vi "Global wiggle variables.vi"() -> ()   [LabVIEW 2017]
panel:
  in  "Z frequency":dbl
  in  "Z amplitude":dbl
  in  "Y frequency":dbl
  in  "Y amplitude":dbl
  out "Wiggle stop":bool
  in  "X frequency":dbl
  in  "X amplitude":dbl
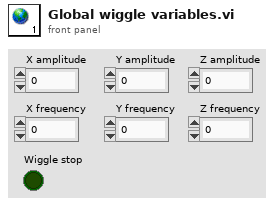
[diagram p1: front panel]
diagram:
